vi "Close.vi"(8 "error in (no error)":errorcluster, 11 "midi file":refnum<class "midi file.lvclass">) -> (0 "error out":errorcluster)   [LabVIEW 2020, in "midi file.lvclass"]
uses:
  midi file.lvclass
  midi file.lvclass/midi file.ctl
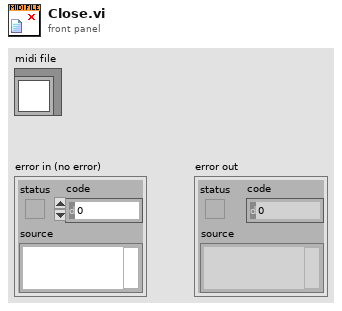
[diagram p1: front panel]
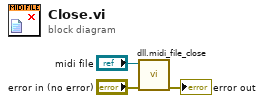
[diagram p0: block diagram]
diagram:
  n1 = call "dll.midi_file_close.vi"("error in (no error)"="error in (no error)", "midi file in"="midi file") -> ("error out"=→"error out":errorcluster)  [unwired: 8 in, 1 out]
